vi "Read FP Control.vi"(8 "error in (no error)":errorcluster, 10 "Control Name":string="Configuration", 11 "Measure Object in":refnum<class "Template Module.lvclass">) -> (0 "error out":errorcluster, 1 "Present":bool, 2 "Control Value":variant, 3 "Measure Object out":refnum<class "Template Module.lvclass">)   [LabVIEW 2016, in "Template Module.lvclass"]
uses:
  Template Module.lvclass
  Template Module.lvclass/Template Module.ctl
  Read Front Panel ref.vi
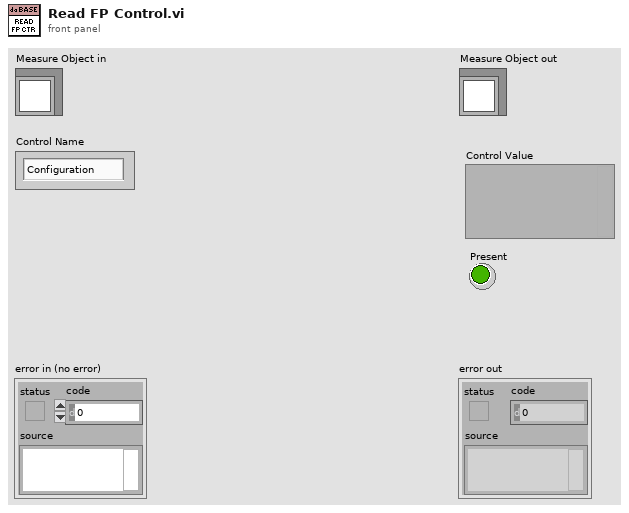
[diagram p1: front panel]
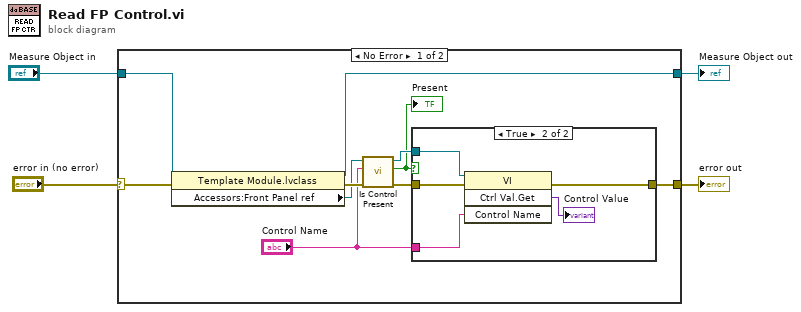
[diagram p0: block diagram]
diagram:
  n1 = case shown="No Error" "error in (no error)" {
    selector: "error in (no error)" -> [w14 w22]
    tunnel: [w11 w22] -> w3
    tunnel: [w12 w21] -> w1
    tunnel: "Measure Object in" -> [w13 w21]
    frame No Error {
      n2 = property class="Template Module.lvclass"(reference=w13, error in=w14) -> (reference out=w12:refnum<class "Template Module.lvclass">, error out=w10:errorcluster, "Accessors:Front Panel ref"=w9:refnum<vi>)
      n3 = call "Is Control Present.vi"("Error In"=w10, "Control label"="Control Name", "VI ref"=w9) -> ("Error Out"=w7:errorcluster, "Present"=w5:bool, "VI ref out"=w8:refnum<vi>)  [unwired: 5 in, 1 out]
      "Present" <- w5
      n4 = case shown="True" w5 {
        tunnel: [w15 w19] -> w11
        tunnel: w8 -> [_ w18]
        tunnel: w7 -> [w15 w17]
        tunnel: "Control Name" -> [_ w16]
        frame False {
        }
        frame True {
          n5 = invoke class="VI" method="Ctrl Val.Get"(reference=w18, error in=w17, "Control Name"=w16) -> (error out=w19:errorcluster, "Get Control Value Variant"=→"Control Value":variant)  [unwired: 1 in, 2 out]
        }
      }
    }
    frame Error {
    }
  }
  "error out" <- w3
  "Measure Object out" <- w1
